vi "smartmeshIP to ni timestamp.vi"(4 "use correction":bool, 6 "set corr due to mismatch in manager time":bool, 10 "microeconds":i32=1025666387, 11 "seconds":i64=1025666387) -> (3 "Dust Timestamp":timestamp)   [LabVIEW 2017]
panel:
  out "correction":dbl format="%#.6f"
  out "x+y":dbl format="%#_6f"
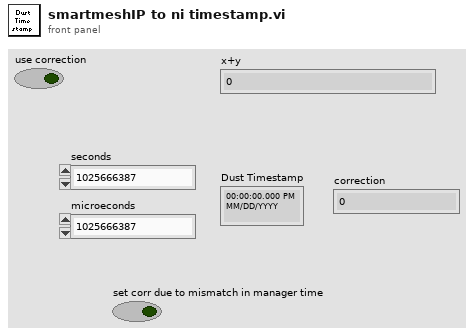
[diagram p1: front panel]
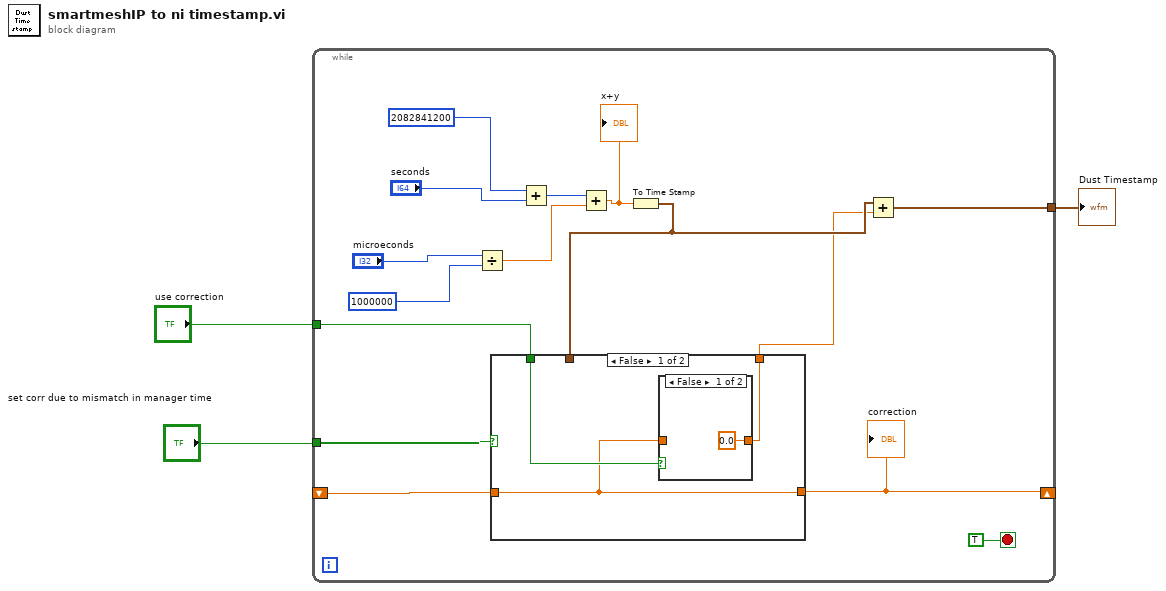
[diagram p0: block diagram]
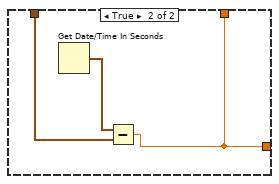
[diagram p3: hidden frame]
diagram:
  n1 = while {
    tunnel: [w8] -> w3
    shift-right: [w5] -> _
    shift-left: _ -> [w10]
    tunnel: "set corr due to mismatch in manager time" -> [w11]
    tunnel: "use correction" -> [w7]
    stop <- TRUE stop-if-true
    n2 = Divide(x="microeconds", y=u32 1000000) -> (x/y=w6:dbl)
    n3 = Add(x=u64 2082841200 ("double precision float 2"), y="seconds") -> (x+y=w15:u64)
    n4 = Add(x=w15, y=w6) -> (x+y=w14:dbl)
    "x+y" <- w14
    n5 = To Time Stamp(1:w14) -> (0:w9:timestamp)
    n6 = case shown="False" w11 {
      tunnel: w9 -> [_ w25]
      tunnel: [w20 w24] -> w5
      tunnel: w10 -> [w20 _]
      tunnel: w7 -> [w21 _]
      tunnel: [w19 w24] -> w4
      frame False {
        n7 = case shown="False" w21 {
          tunnel: [0.0 w23] -> w19
          tunnel: w20 -> [_ w23]
          frame False {
          }
          frame True {
          }
        }
      }
      frame True {
        n8 = Get Date/Time In Seconds() -> (seconds since 1Jan1904=w26:timestamp)
        n9 = Subtract(x=w26, y=w25) -> (x-y=w24:dbl)
      }
    }
    "correction" <- w5
    n10 = Add(x=w9, y=w4) -> (x+y=w8:timestamp)
  }
  "Dust Timestamp" <- w3
